vi "Initialize.vi"(8 "error in":errorcluster, 10 "parameters":variant, 11 "node in":refnum<class "RIO Target.lvclass">) -> (0 "error out":errorcluster, 2 "summary":T2[](array[typedef]), 3 "data value reference":T1)   [LabVIEW 2014, in "RIO Target.lvclass"]
doc: "Initializes the data of a node to its default state.\nThe object is not created inside of this VI, because it is created from a File depending on user selection."
uses:
  RIO Target.lvclass
  <vilib>/NI/Configuration Framework/Node/Summary.ctl
  <vilib>/NI/Configuration Framework/Node/NodeRef.ctl
  <vilib>/NI/Configuration Framework/Node/NISE_CEF_Node.lvclass
  RIO Target Configuration/RIO Target Configuration.lvclass
  <vilib>/NI/Configuration Framework/serializable configuration/set metadata property.vi
  <vilib>/NI/Configuration Framework/serializable node/NISE_CEF_serializable node.lvclass
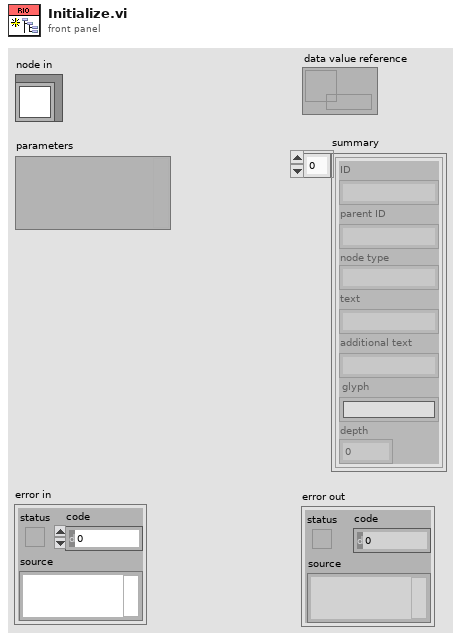
[diagram p1: front panel]
types:
  T1 = typedef "NISE_CEF_Node.lvclass/NodeRef.ctl" = refnum<data-value>
  T2 = typedef "NISE_CEF_Node.lvclass/Summary.ctl" = cluster{"ID":string, "parent ID":string, "node type":string, "text":string, "additional text":string, "glyph":string, "depth":i32}
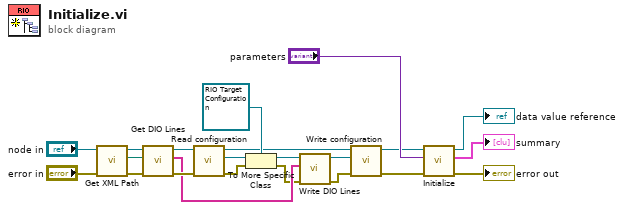
[diagram p0: block diagram]
diagram:
  n1 = call-dynamic "Get XML Path.vi"("error in (no error)"="error in", "RIO Target in"="node in") -> ("error out"=w19:errorcluster, "XML Path"=w20:path, "RIO Target out"=w21:refnum<class "RIO Target.lvclass">)  [unwired: 7 in]
  n2 = call "Get DIO Lines.vi"("error in (no error)"=w19, "path to XML document"=w20, "RIO Target in"=w21) -> ("error out"=w12:errorcluster, "DIO Lines"=w11:string[], "RIO Target out"=w16:refnum<class "RIO Target.lvclass">)  [unwired: 6 in]
  n3 = call-dynamic "Read configuration.vi"("error in"=w12, "RIO Target in"=w16) -> ("error out"=w10:errorcluster, "configuration"=w15:refnum<class "NISE_CEF_serializable configuration.lvclass">, "RIO Target out"=w7:refnum<class "RIO Target.lvclass">)  [unwired: 7 in]
  n4 = To More Specific Class(target class=refnum<class "RIO Target Configuration.lvclass"> refnum ("RIO Target Configuration in"), reference=w15, error in=w10) -> (specific class reference=w13:refnum<class "RIO Target Configuration.lvclass">, error out=w9:errorcluster)
  n5 = call "Write DIO Lines.vi"("error in (no error)"=w9, "DIO Lines"=w11, "RIO Target Configuration in"=w13) -> ("error out"=w8:errorcluster, "RIO Target Configuration out"=w6:refnum<class "RIO Target Configuration.lvclass">)  [unwired: 7 in]
  n6 = call-dynamic "Write configuration.vi"("error in"=w8, "configuration"=w6, "RIO Target in"=w7) -> ("error out"=w4:errorcluster, "RIO Target out"=w5:refnum<class "RIO Target.lvclass">)  [unwired: 7 in]
  n7 = call-parent "Initialize.vi"("error in"=w4, "parameters"="parameters", "node in"=w5) -> ("error out"=→"error out":errorcluster, "summary"=→"summary":T2[], "data value reference"=→"data value reference":T1)  [unwired: 6 in]
